vi "1830C Commands.vi"(0 "Instrument Resource Name":refnum<visa-resource-name>, 7 "Command":u16(ring) items=["Attenuator OFF", "Attenuator ON", "Attenuator Query", "Beep OFF", "Beep ON", "Beep Query", "Clear Status Reg", "Data Query (nW)", "Echo OFF", "Echo ON", "Echo Query", "FIlter Slow", "Filter Medium", "Filter Fast", "Filter Query", "Hold", "Go", "Go Query", "Backlight OFF", "Backlight Medium", "Backlight High", "Backlight Query", "Local Lockout OFF", "Local Lockout ON", "Local Lockout Query", "Service Request Enable", "Service Request Query", "Auto Callibration", "Status Regiater Query", "Auto Range", "Signal Range 1", "Signal Range 2", "Signal Range 3", "Signal Range 4", "Signal Range 5", "Signal Range 6", "Signal Range 7", "Signal Range 8", "Signal Range Query", "Store Reference", "Units W", "Units dB", "Units dBm", "Units REL", "Units Query", "Set Wavelength", "Wavelength Querry", "Zero OFF", "Zero ON", "Zero Query"], 9 "Wavelength":string, 11 "error in (no error)":errorcluster, 12 "Range":bool) -> (4 "VISA resource name out":refnum<visa-resource-name>, 8 "LM Response":dbl format="%#_4f", 15 "error out":errorcluster {"code" format="%.0x"})   [LabVIEW 2010]
uses:
  <vilib>/Instr/_visa.llb/VISA Configure Serial Port (Instr).vi
panel:
  out "Numeric":dbl
  out "Bytes Read":dbl
  out "Read String":string
  in  "Serial Configuration":T1={"Baud Rate"=9600, "Parity"=0, "Data Bits"=7, "Stop Bits"=10, "Flow Control"=0} {"Flow Control" items=["None", "XON/XOFF", "RTS/CTS", "XON/XOFF & RTS/CTS", "DTR/DSR", "XON/XOFF & DTR/DSR"]; "Stop Bits" items=["1.0"=10, "1.5"=15, "2.0"=20]; "Data Bits" items=["7"=7, "8"=8]; "Parity" items=["None", "Odd", "Even", "Mark", "Space"]; "Baud Rate" items=["300"=300, "600"=600, "1200"=1200, "2400"=2400, "4800"=4800, "9600"=9600, "19200"=19200]}
  # "Nano"
  # "Pico"
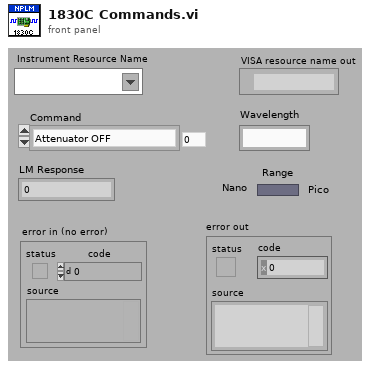
[diagram p1: front panel]
types:
  T1 = cluster{"Baud Rate":u32, "Parity":u16, "Data Bits":u16, "Stop Bits":u16, "Flow Control":u16}
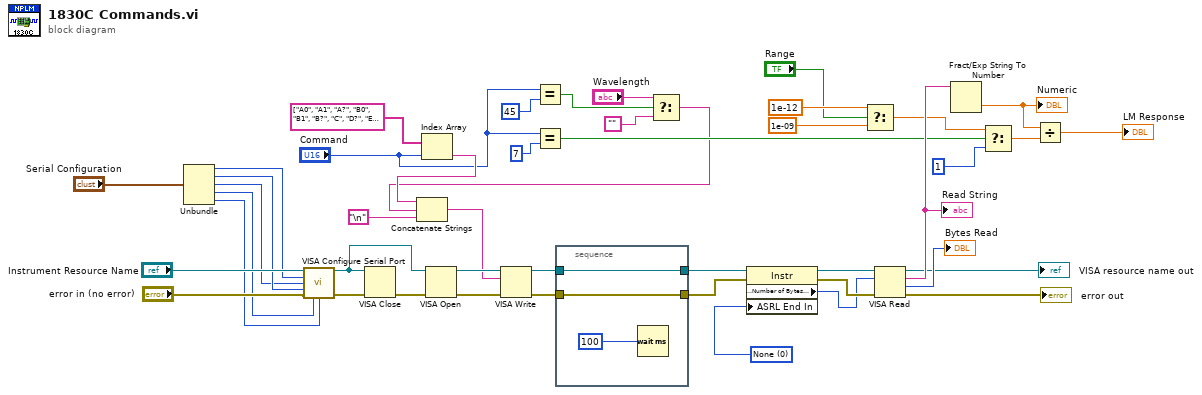
[diagram p0: block diagram]
diagram:
  w30 = u16 0 items=["None", "LastBit", "TermChar"] ("Serial Settings:Serial End Mode for Reads")
  n1 = Unbundle("Serial Configuration") -> ("Baud Rate"=w39:u32, "Parity"=w38:u16, "Data Bits"=w37:u16, "Stop Bits"=w36:u16, "Flow Control"=w35:u16)
  n2 = call-poly "VISA Configure Serial Port"("VISA resource name"="Instrument Resource Name", "baud rate (9600)"=w39, "data bits (8)"=w37, "parity (0:none)"=w38, "error in (no error)"="error in (no error)", "stop bits (10: 1 bit)"=w36, "flow control (0:none)"=w35) -> ("VISA resource name out"=w44:refnum<visa-resource-name>, "error out"=w43:errorcluster)  [unwired: 7 in]
  n3 = VISA Close(VISA resource name=w44, error in (no error)=w43) -> (error out=w45:errorcluster)
  n4 = Index Array(array=string[] ["A0", "A1", "A?", "B0", "B1", "B?", "C", "D?", "E0", "E1", "E?", "F1\nF1", "F2", "F3", "F?", "G0", "G1", "G?", "K0", "K1", "K2", "K?", "L0", "L1", "L?", "M", "M?", "O", "Q?", "R0", "R1", "R2", "R3", "R4", "R5", "R6", "R7", "R8", "R?", "S", "U1", "U2", "U3", "U4", "U?", "W", "W?", "Z0", "Z1", "Z?"], index="Command") -> (element=w18:string)
  n5 = VISA Open(error in (no error)=w45, VISA resource name=w44) -> (VISA resource name=w34:refnum<visa-resource-name>, error out=w33:errorcluster)  [unwired: 3 in]
  n6 = Equal?(x="Command", y=45) -> (x = y?=w8:bool)
  n7 = Equal?(x="Command", y=7) -> (x = y?=w14:bool)
  n8 = Select(t="Wavelength", s=w8, f="") -> (s? t:f=w7:string)
  n9 = Concatenate Strings(w18, w7, "\n") -> (w28:string)
  n10 = VISA Write(VISA resource name=w34, write buffer=w28, error in (no error)=w33) -> (VISA resource name out=w26:refnum<visa-resource-name>, error out=w24:errorcluster)  [unwired: 1 out]
  n11 = stacked-sequence {
    tunnel: w26 -> [w48]
    tunnel: [w48] -> w25
    tunnel: [w47] -> w23
    tunnel: w24 -> [w47]
    frame #0 {
      n12 = Wait (ms)(milliseconds to wait=u32 100 ("delay before read (ms)")) -> ()  [unwired: 1 out]
    }
  }
  n13 = property class="Instr"(reference=w25, error in=w23, "ASRL End In"=w30) -> (reference out=w32:refnum<visa-resource-name>, error out=w31:errorcluster, "Serial Settings:Number of Bytes at Serial Port"=w27:u32)
  n14 = Select(t=1e-12, s="Range", f=1e-09) -> (s? t:f=w4:dbl)
  n15 = VISA Read(VISA resource name=w32, byte count=w27, error in (no error)=w31) -> (VISA resource name out=→"VISA resource name out":refnum<visa-resource-name>, read buffer=w22:string, return count=→"Bytes Read":u32, error out=→"error out":errorcluster)
  "Read String" <- w22
  n16 = Fract/Exp String To Number(string=w22) -> (number=w21:dbl)  [unwired: 3 in, 1 out]
  "Numeric" <- w21
  n17 = Select(t=w4, s=w14, f=1) -> (s? t:f=w17:dbl)
  n18 = Divide(x=w21, y=w17) -> (x/y=→"LM Response":dbl)
